vi "Analysatoren abgleichen Ring.vi"(10 "Strings und Werte []":T1 caption="Ring Strings und Werte []", 11 "Strings und Werte []":cluster{"String":string, "Value":string}[](array[cluster])) -> (3 "x != y?":bool)   [LabVIEW 2020, in "System Einstellungen V2.lvlib"]
uses:
  System Einstellungen V2.lvlib
  <vilib>/Utility/miscctls.llb/LVStringsAndValuesArrayTypeDef_U16.ctl
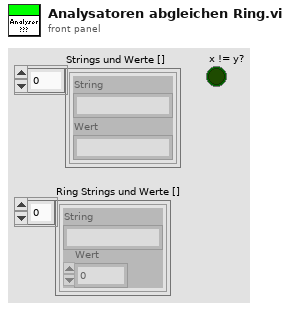
[diagram p1: front panel]
types:
  T1 = typedef "LVStringsAndValuesArrayTypeDef_U16.ctl" = cluster{"String":string, "Value":u16}[]
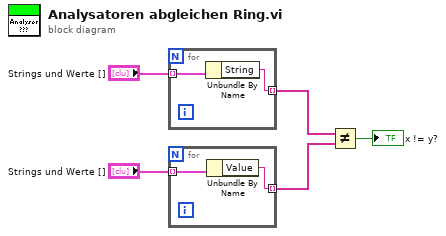
[diagram p0: block diagram]
diagram:
  n1 = for {
    tunnel: [w6] -> w5 mode=indexing
    tunnel: "Strings und Werte []" -> [w7] mode=indexing
    n2 = Unbundle By Name(w7) -> ("String"=w6:string)
  }
  n3 = for {
    tunnel: [w8] -> w2 mode=indexing
    tunnel: "Strings und Werte []" -> [w9] mode=indexing
    n4 = Unbundle By Name(w9) -> ("Value"=w8:string)
  }
  n5 = Not Equal?(x=w5, y=w2) -> (x != y?=→"x != y?":bool)
